vi "enable.vi"(7 "Error In":errorcluster, 10 "Modbus master in":refnum<class "Modbus Master.lvclass">) -> (0 "Error Out":errorcluster, 3 "Modbus master out":refnum<class "Modbus Master.lvclass">)   [LabVIEW 2019]
uses:
  <vilib>/NI/Modbus Library/API/Master/Modbus Master.lvclass
  controls/holdingRegistersNames.ctl
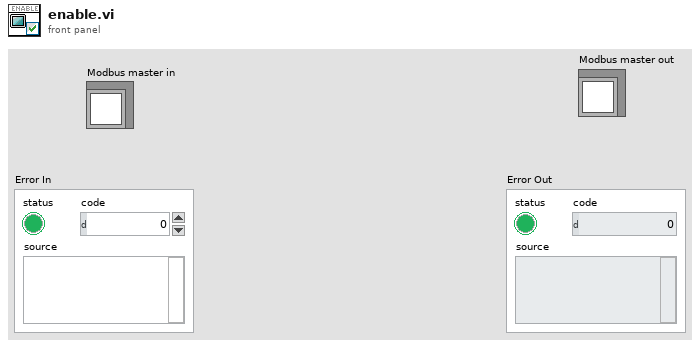
[diagram p1: front panel]
types:
  T1 = typedef "holdingRegistersNames.ctl" = u16
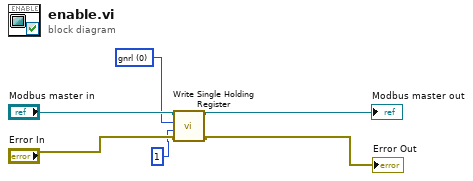
[diagram p0: block diagram]
diagram:
  w1 = T1 0 items=["gnrl", "startCmd", "fillingPotInd", "porFilledInd", "fillPotCmd", "TankDrainCmd", ""] ("Text Ring")
  n1 = call-dynamic "Write Single Holding Register.vi"("error in"="Error In", "register to write"=u16 1 ("number of inputs"), "address"=w1, "Modbus master in"="Modbus master in") -> ("error out"=→"Error Out":errorcluster, "Modbus master out"=→"Modbus master out":refnum<class "Modbus Master.lvclass">)  [unwired: 6 in]
